vi "Normalize.vi"   [LabVIEW 2020, in "NI_AALBase.lvlib"]
doc: "Normalizes the input vector or matrix using its statistical profile (micro,s), where micro is the <B>mean</B> and s is the <B>standard deviation</B>, to obtain a <B>Normalized Vector</B> or <B>Normalized Matrix</B> whose statistical profile is (0,1)."
uses:
  NI_AALBase.lvlib
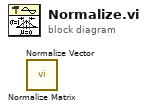
[diagram p0: block diagram]
diagram:
  n1 = call "Normalize Matrix.vi"() -> ()  [unwired: 2 in, 4 out]
  n2 = call "Normalize Vector.vi"() -> ()  [unwired: 2 in, 4 out]
